vi "Sender.vi"() -> ()   [LabVIEW 2019]
uses:
  <vilib>/Platform/TimedLoop/XDataNode/timing_clust.ctl
  <vilib>/Platform/TimedLoop/XDataNode/nitl_modes.ctl
  <vilib>/Platform/TimedLoop/XDataNode/wakeup.ctl
  <vilib>/platform/TimedLoop/XDataNode/XDataNode.xnode
  <vilib>/Platform/TimedLoop/XDataNode/XDNodeRunTimeDep.lvlib
panel:
  out "index":i32
  out "open error":errorcluster
  out "write error":errorcluster
  out "open status":bool
  in  "Stop":bool
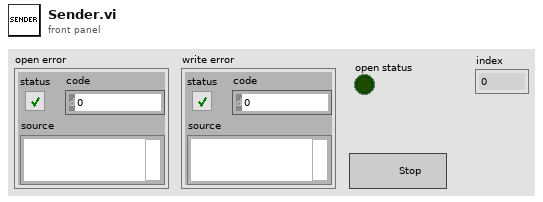
[diagram p1: front panel]
types:
  T1 = typedef "XDNodeRunTimeDep.lvlib/timing_clust.ctl" = cluster{"Expected End [f-1]":u64, "Actual End [f-1]":u64, "Finished Late? [f-1]":bool, "Expected End [i-1]":u64, "Actual End [i-1]":u64, "Finished Late? [i-1]":bool, "Expected Start [i]":u64, "Actual Start [i]":u64, "Expected Start [f]":u64, "Actual Start [f]":u64, "Source Name":string, "Structure Name":string, "Period":i64, "Deadline":i64, "Offset":i64, "Start":i64, "Priority":i32, "Timeout":i32, "Mode":T2, "Wakeup Reason":T3, "Error":errorcluster, "Source Type":string, "Secondary Source Type":string, "Global End Time":u64, "Global Start Time":u64, "Frame Duration":u64, "Iteration Duration":u64, "Assigned CPU":i32, "I/O Scan Engine Mode":u32}
  T2 = typedef "XDNodeRunTimeDep.lvlib/nitl_modes.ctl" = enum32{"No Change", "Process missed periods, maintain original phase", "Discard missed periods, maintain original phase", "Process missed periods, ignore original phase", "Discard missed periods, ignore original phase"}
  T3 = typedef "XDNodeRunTimeDep.lvlib/wakeup.ctl" = enum32{"Normal", "Aborted", "Asynchronous wakeup", "Timing source error", "Timed loop error", "Timeout"}
  T4 = typedef "Data.ctl" = cluster{"P_DUT":dbl, "P_Chamber":dbl}
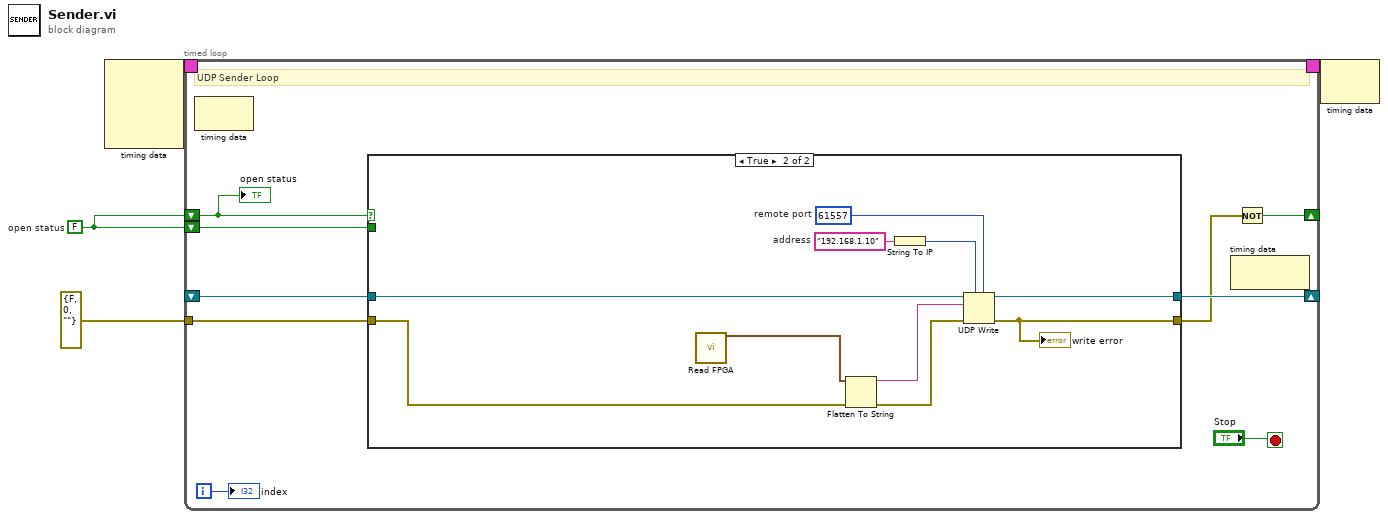
[diagram p0: block diagram]
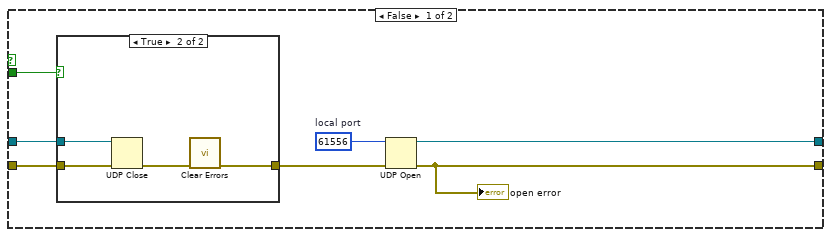
[diagram p2: hidden frame]
diagram:
  w1 = FALSE  # open status
  n1 = node-c288() -> (w4:T1)  [unwired: 4 in]
  n2 = timed-loop {
    tunnel: errorcluster {"status"=FALSE, "code"=0, "source"=""} ("error out") -> [w12]
    timing: w4 -> [_]
    timing-out: [_] -> w3
    shift-right: [w10] -> _
    shift-left: _ -> [w13]
    shift-right: [w6] -> _
    shift-left: w1 -> [w9]
    shift-left: w1 -> [w8]
    i -> [w5]
    stop <- "Stop" stop-if-true
    # "UDP Sender Loop"
    n3 = node-c288() -> ()  [unwired: 1 in, 1 out]
    n4 = case shown="True" w9 {
      tunnel: w13 -> [w19 w35]
      tunnel: w12 -> [w18 w27]
      tunnel: [w15 w34] -> w10
      tunnel: [w14 w33] -> w7
      tunnel: w8 -> [w17 _]
      frame False {
        w20 = u16 61556  # local port
        n5 = case shown="True" w17 {
          tunnel: w19 -> [_ w25]
          tunnel: w18 -> [w21 w24]
          tunnel: [w21 w22] -> w16
          frame False {
          }
          frame True {
            n6 = UDP Close(connection ID=w25, 8:w24) -> (error out=w23:errorcluster)  [unwired: 1 out]
            n7 = call <vilib>:"Clear Errors.vi"("error in (no error)"=w23) -> ("error out"=w22:errorcluster)  [unwired: 5 in, 1 out]
          }
        }
        n8 = UDP Open(8:w16, 11:w20) -> (port=w15:refnum<k16>, 0:w14:errorcluster)  [unwired: 3 in, 1 out]
        "open error" <- w14
      }
      frame True {
        w31 = "192.168.1.10"  # address
        w32 = u16 61557  # remote port
        n9 = call "Read FPGA.vi"() -> ("Data"=w28:T4)  [unwired: 15 in]
        n10 = Flatten To String(anything=w28, error in (no error)=w27) -> (data string=w29:string, error out=w26:errorcluster)  [unwired: 2 in, 1 out]
        n11 = String To IP(1:w31) -> (0:w30:u32)
        n12 = UDP Write(address=w30, port or service name=w32, connection ID=w35, data in=w29, 8:w26) -> (error out=w33:errorcluster, 3:w34:refnum<k16>)  [unwired: 1 in]
        "write error" <- w33
      }
    }
    n13 = node-c288() -> ()  [unwired: 1 in, 1 out]
    n14 = Not(x=w7) -> (.not. x?=w6:bool)
    "open status" <- w9
    "index" <- w5
  }
  n15 = node-c288(w3) -> ()  [unwired: 1 out]
